vi "Joystick control with DEADBAND, LIMITS, and MIN.vi"(4 "slow?":bool, 6 "Parameters":T1={"MAX LIMIT"=0.8, "MIN SPEED"=0.25, "DEADBAND"=0.05, "invert X?"=FALSE, "invert Y?"=FALSE} {"DEADBAND" format="%#_13g"; "MIN SPEED" format="%#_13g"; "MAX LIMIT" format="%#_13g"}, 8 "TURBO?":bool, 10 "Joystick Y":dbl(slide) min=-1.0 max=1.0 step=0.05 scale=-1.0..1.0 scale format="%.3f", 11 "Joystick X":dbl(slide) min=-1.0 max=1.0 step=0.05 scale=-1.0..1.0 scale format="%.3f") -> (0 "polar out":cluster{"R":dbl, "deg":dbl} {"R" format="%.3f"; "deg" format="%.3f"}, 2 "Y out":dbl format="%.3f", 3 "X out":dbl format="%.3f")   [LabVIEW 2019]
uses:
  <vilib>/Analysis/coordinate.llb/3D Coordinate Conversion (Scalar).vi
  <vilib>/Analysis/NI_AALPro.lvlib
panel:
  in  "invert Y?":bool
  in  "invert X?":bool
  in  "MIN":dbl=0.3 format="%#_13g"
  in  "MAX LIMIT":dbl=0.8 format="%#_13g"
  in  "DEADBAND":dbl=0.1 format="%#_13g"
  in  "TESTING":bool
  in  "stop":bool
  # "Minimum output value when axis is = DEADBAND;\naxis value of DEADBAND to 1 is scaled across MIN \nto MAX"
  # "Maximum output value IF TURBO? toggle is OFF;\nmax output goes to 1 if TURBO? is ON."
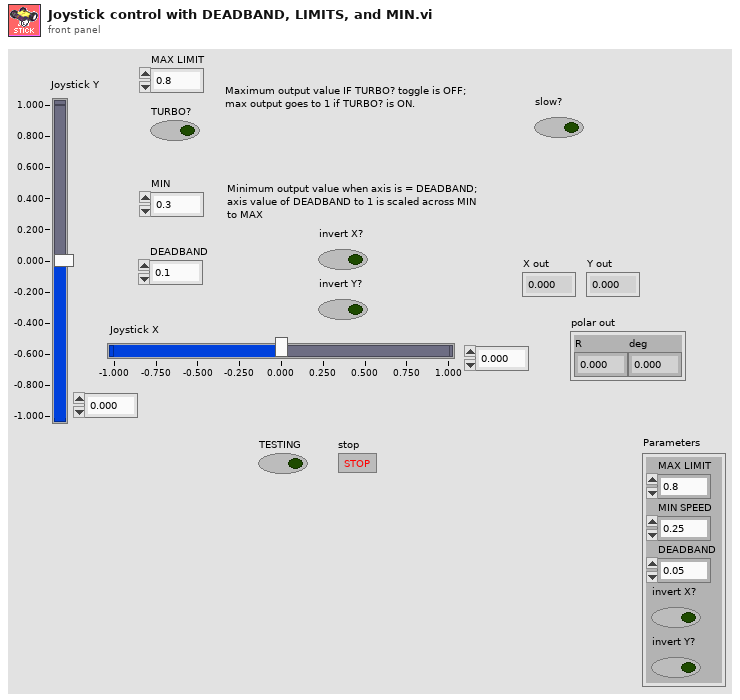
[diagram p1: front panel]
types:
  T1 = cluster{"MAX LIMIT":dbl, "MIN SPEED":dbl, "DEADBAND":dbl, "invert X?":bool, "invert Y?":bool}
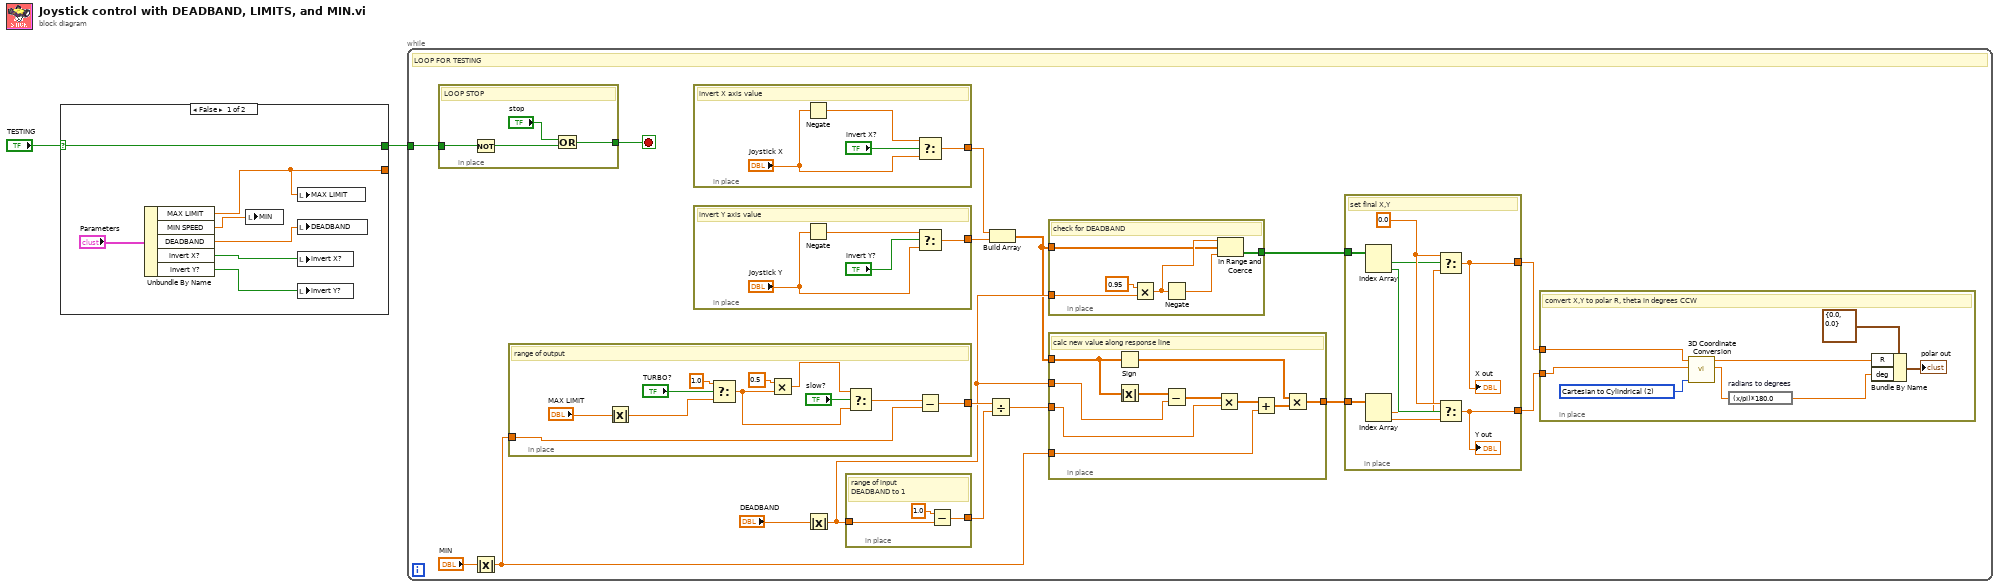
[diagram p0: block diagram]
diagram:
  n1 = case shown="False" "TESTING" {
    selector: "TESTING" -> [w9 w10]
    tunnel: [w9 w10] -> w1
    tunnel: [w5 _] -> _
    frame False {
      n2 = Unbundle By Name("Parameters") -> ("MAX LIMIT"=w5:dbl, "MIN SPEED"=w7:dbl, "DEADBAND"=w6:dbl, "invert X?"=w4:bool, "invert Y?"=w3:bool)
      n3 = local write "MIN"(w7) -> ()
      n4 = local write "MAX LIMIT"(w5) -> ()
      n5 = local write "DEADBAND"(w6) -> ()
      n6 = local write "invert X?"(w4) -> ()
      n7 = local write "invert Y?"(w3) -> ()
    }
    frame True {
    }
  }
  n8 = while {
    tunnel: w1 -> [w24]
    stop <- w26 stop-if-true
    # "LOOP FOR TESTING"
    n9 = in-place {
      in-place-border: [w84] -> w26
      in-place-border: w24 -> [w82]
      # "LOOP STOP"
      n10 = Not(x=w82) -> (.not. x?=w83:bool)
      n11 = Or(x="stop", y=w83) -> (x .or. y?=w84:bool)
    }
    n12 = Absolute Value(x="MIN") -> (abs(x)=w16:dbl)
    n13 = in-place {
      in-place-border: w16 -> [w75]
      in-place-border: [w74] -> w25
      # "range of output"
      n14 = Absolute Value(x="MAX LIMIT") -> (abs(x)=w68:dbl)
      n15 = Select(t=1.0, s="TURBO?", f=w68) -> (s? t:f=w69:dbl)
      n16 = Multiply(x=0.5 ("t"), y=w69) -> (x*y=w70:dbl)
      n17 = Select(t=w70, s="slow?", f=w69) -> (s? t:f=w73:dbl)
      n18 = Subtract(x=w73, y=w75) -> (x-y=w74:dbl)
    }
    n19 = in-place {
      in-place-border: [w67] -> w18
      # "invert X axis value"
      n20 = Negate(x="Joystick X") -> (-x=w65:dbl)
      n21 = Select(t=w65, s="invert X?", f="Joystick X") -> (s? t:f=w67:dbl)
    }
    n22 = in-place {
      in-place-border: [w63] -> w17
      # "invert Y axis value"
      n23 = Negate(x="Joystick Y") -> (-x=w61:dbl)
      n24 = Select(t=w61, s="invert Y?", f="Joystick Y") -> (s? t:f=w63:dbl)
    }
    n25 = Absolute Value(x="DEADBAND") -> (abs(x)=w14:dbl)
    n26 = in-place {
      in-place-border: w14 -> [w80]
      in-place-border: [w79] -> w23
      # "range of input \nDEADBAND to 1"
      n27 = Subtract(x=1.0, y=w80) -> (x-y=w79:dbl)
    }
    n28 = Divide(x=w25, y=w23) -> (x/y=w15:dbl)
    n29 = Build Array(w18, w17) -> (w12:dbl[])
    n30 = in-place {
      in-place-border: [w58] -> w11
      in-place-border: w12 -> [w55]
      in-place-border: w14 -> [w54]
      # "check for DEADBAND"
      n31 = Multiply(x=0.95, y=w54) -> (x*y=w57:dbl)
      n32 = Negate(x=w57) -> (-x=w59:dbl)
      n33 = In Range and Coerce(upper limit=w57, x=w55, lower limit=w59) -> (In Range?=w58:bool[])  [unwired: 1 out]
    }
    n34 = in-place {
      in-place-border: w12 -> [w53]
      in-place-border: w16 -> [w49]
      in-place-border: w15 -> [w48]
      in-place-border: w14 -> [w47]
      in-place-border: [w44] -> w13
      # "calc new value along response line"
      n35 = Sign(1:w53) -> (0:w45:dbl[])
      n36 = Absolute Value(x=w53) -> (abs(x)=w52:dbl[])
      n37 = Subtract(x=w52, y=w47) -> (x-y=w51:dbl[])
      n38 = Multiply(x=w51, y=w48) -> (x*y=w50:dbl[])
      n39 = Add(x=w50, y=w49) -> (x+y=w46:dbl[])
      n40 = Multiply(x=w45, y=w46) -> (x*y=w44:dbl[])
    }
    n41 = in-place {
      in-place-border: [w42] -> w20
      in-place-border: [w41] -> w19
      in-place-border: w13 -> [w37]
      in-place-border: w11 -> [w38]
      w43 = 0.0 ("t")
      # "set final X,Y"
      n42 = Index Array(array=w38) -> (element #1=w40:bool, element #2=w39:bool)  [unwired: 2 in]
      n43 = Index Array(array=w37) -> (element #1=w36:dbl, element #2=w35:dbl)  [unwired: 2 in]
      n44 = Select(t=w43, s=w40, f=w36) -> (s? t:f=w42:dbl)
      "X out" <- w42
      n45 = Select(t=w43, s=w39, f=w35) -> (s? t:f=w41:dbl)
      "Y out" <- w41
    }
    n46 = in-place {
      in-place-border: w20 -> [w34]
      in-place-border: w19 -> [w33]
      w32 = u16 2 items=["Cartesian to Spherical", "Spherical to Cartesian", "Cartesian to Cylindrical", "Cylindrical to Cartesian", "Spherical to Cylindrical", "Cylindrical to Spherical"] ("conversion type")
      # "convert X,Y to polar R, theta in degrees CCW"
      n47 = call-poly <vilib>:"3D Coordinate Conversion.vi"("conversion type"=w32, "axis 2"=w33, "axis 1"=w34) -> ("axis 2 out"=w29:dbl, "axis 1 out"=w30:dbl)  [unwired: 5 in, 2 out]
      n48 = expression code="(x/pi)*180.0" "radians to degrees"(w29) -> (w28:dbl)
      n49 = Bundle By Name(cluster=cluster{"R":dbl, "deg":dbl} {"R"=0.0, "deg"=0.0}, "R"=w30, "deg"=w28) -> (→"polar out":cluster{"R":dbl, "deg":dbl})
    }
  }
